vi "LJstreamUD read config.vi"(0 "Working Directory":path, 5 "filename":string="ljstreamud.cfg", 7 "ChP Default":string="0#!#1#!#2#!#3#!#4#!#5#!#6#!#7#!#8#!#9#!#10#!#11#!#12#!#13#!#14#!#15#!#") -> (1 "Data File Prefix":string="data", 2 "Scan Rate (Hz)":dbl=500.0 format="%.3f", 3 "Graph History":i32=1000 min=0, 4 "# Channels":i32=4, 6 "Disable Scaling":bool, 8 "Max File Size (Bytes)":i32=1048576, 9 "Write To File":bool, 10 "Channel Setup":T1={"+Ch"=["0", "1", "2", "3", "4", "5", "6", "7"], "-Ch"=["199", "199", "199", "199", "199", "199", "199", "199"], "Ranges"=[0, 0, 0, 0, 0, 0, 0, 0], "Scaling Equation"=["y=v0", "y=v1", "y=v2", "y=v3", "y=v4", "y=v5", "y=v6", "y=v7"], "Graph?"=[]} {"Ranges" items=["LJ_rgBIP10V", "LJ_rgBIP5V", "LJ_rgUNI5V", "LJ_rgUNI2P5V", "LJ_rgUNI1P25V", "LJ_rgBIP1V", "LJ_rgUNIP625V", "LJ_rgBIPP1V", "LJ_rgBIPP01V"]}, 12 "Interval (ms)":u32=500, 13 "Resolution":u8, 14 "SettlingFactor":u8, 15 "error out":errorcluster)   [LabVIEW 2021]
uses:
  <vilib>/Utility/config.llb/Read Key (String).vi
  <vilib>/Utility/config.llb/Read Key (U32).vi
  <vilib>/Utility/config.llb/Read Key (Double).vi
  <vilib>/Utility/config.llb/Read Key (I32).vi
  <vilib>/Utility/config.llb/Read Key (Boolean).vi
  <vilib>/Utility/config.llb/NI_LVConfig.lvlib
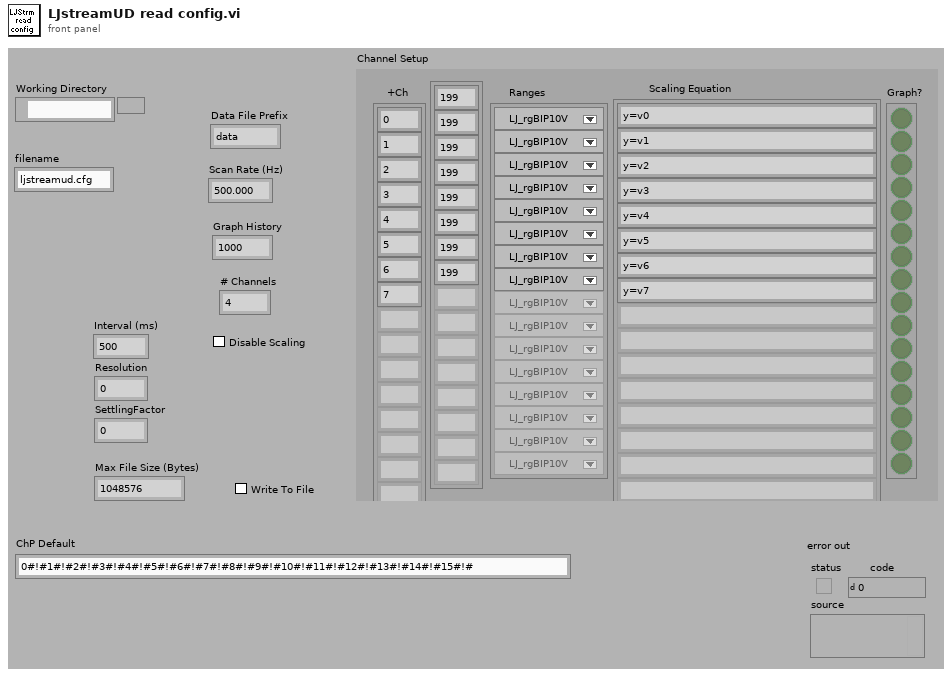
[diagram p1: front panel]
types:
  T1 = cluster{"+Ch":string[], "-Ch":string[], "Ranges":u16[], "Scaling Equation":string[], "Graph?":bool[]}
  T2 = typedef "NI_LVConfig.lvlib/Config Data RefNum.ctl" = refnum<k1>
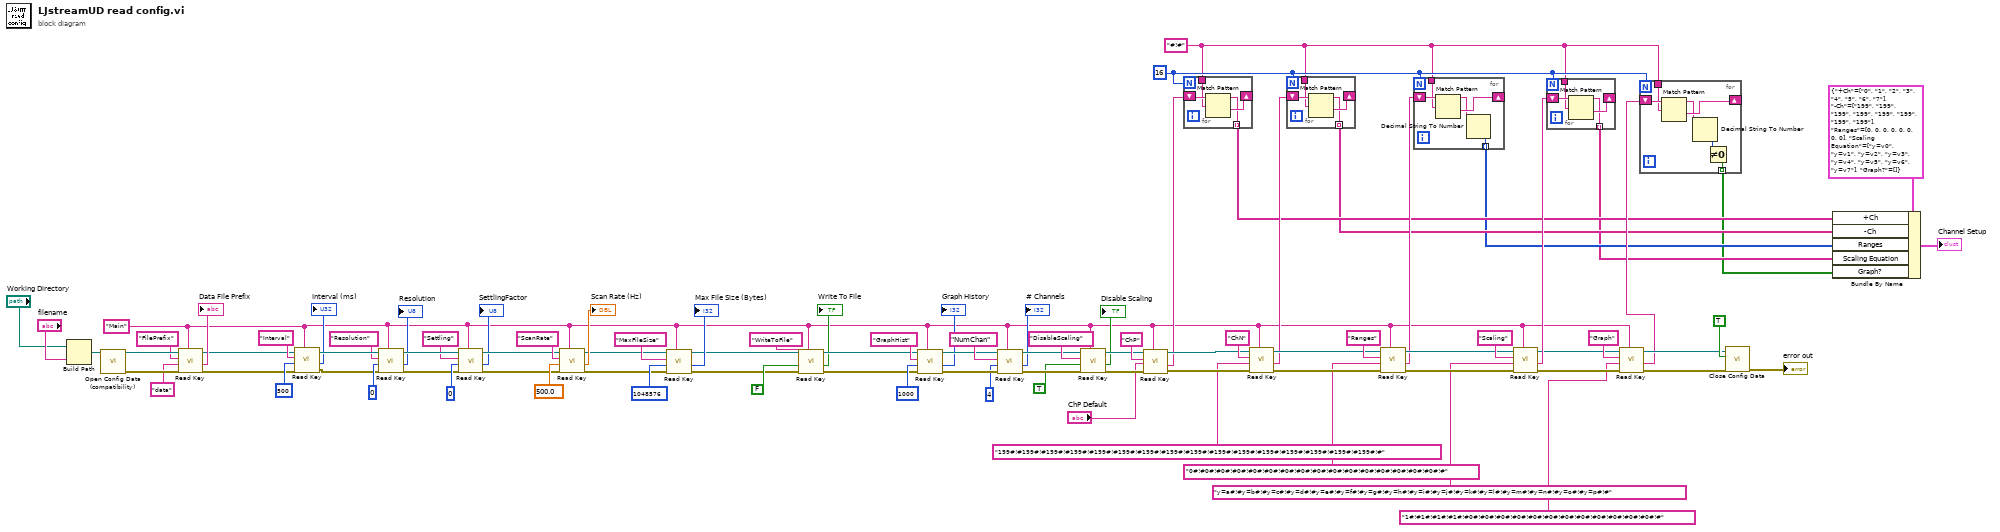
[diagram p0: block diagram]
diagram:
  w50 = 16
  w48 = "#!#" ("delimiter (Tab)")
  w1 = "Main" ("section")
  n1 = Build Path(base path="Working Directory", name or relative path="filename") -> (appended path=w91:path)
  n2 = call <vilib>:"Open Config Data (compatibility).vi"("configuration file path"=w91) -> ("error out"=w88:errorcluster, "refnum"=w89:T2)  [unwired: 8 in, 1 out]
  n3 = call-poly <vilib>:"Read Key.vi"("section"=w1, "error in (no error)"=w88, "default value"="data" ("Data File Prefix"), "key"="FilePrefix", "refnum"=w89) -> ("error out"=w22:errorcluster, "value"=→"Data File Prefix":string, "refnum out"=w20:T2)  [unwired: 3 in, 1 out]
  n4 = call-poly <vilib>:"Read Key.vi"("section"=w1, "error in (no error)"=w22, "default value"=u32 500 ("Scan Rate (Hz)"), "key"="Interval", "refnum"=w20) -> ("error out"=w27:errorcluster, "value"=→"Interval (ms)":u32, "refnum out"=w26:T2)  [unwired: 3 in, 1 out]
  n5 = call-poly <vilib>:"Read Key.vi"("section"=w1, "error in (no error)"=w27, "default value"=u8 0 ("Graph History"), "key"="Resolution", "refnum"=w26) -> ("error out"=w29:errorcluster, "value"=→"Resolution":u32, "refnum out"=w28:T2)  [unwired: 3 in, 1 out]
  n6 = call-poly <vilib>:"Read Key.vi"("section"=w1, "error in (no error)"=w29, "default value"=u8 0 ("# Channels"), "key"="Settling", "refnum"=w28) -> ("error out"=w21:errorcluster, "value"=→"SettlingFactor":u32, "refnum out"=w19:T2)  [unwired: 3 in, 1 out]
  n7 = call-poly <vilib>:"Read Key.vi"("section"=w1, "error in (no error)"=w21, "default value"=500.0 ("Scan Rate (Hz)"), "key"="ScanRate", "refnum"=w19) -> ("error out"=w12:errorcluster, "value"=→"Scan Rate (Hz)":dbl, "refnum out"=w11:T2)  [unwired: 3 in, 1 out]
  n8 = call-poly <vilib>:"Read Key.vi"("section"=w1, "error in (no error)"=w12, "default value"=1048576 ("Graph History"), "key"="MaxFileSize", "refnum"=w11) -> ("error out"=w5:errorcluster, "value"=→"Max File Size (Bytes)":i32, "refnum out"=w6:T2)  [unwired: 3 in, 1 out]
  n9 = call-poly <vilib>:"Read Key.vi"("section"=w1, "error in (no error)"=w5, "default value"=FALSE, "key"="WriteToFile", "refnum"=w6) -> ("error out"=w3:errorcluster, "value"=→"Write To File":bool, "refnum out"=w4:T2)  [unwired: 3 in, 1 out]
  n10 = call-poly <vilib>:"Read Key.vi"("section"=w1, "error in (no error)"=w3, "default value"=1000 ("Graph History"), "key"="GraphHist", "refnum"=w4) -> ("error out"=w83:errorcluster, "value"=→"Graph History":i32, "refnum out"=w84:T2)  [unwired: 3 in, 1 out]
  n11 = call-poly <vilib>:"Read Key.vi"("section"=w1, "error in (no error)"=w83, "default value"=4 ("# Channels"), "key"="NumChan", "refnum"=w84) -> ("error out"=w58:errorcluster, "value"=→"# Channels":i32, "refnum out"=w59:T2)  [unwired: 3 in, 1 out]
  n12 = call-poly <vilib>:"Read Key.vi"("section"=w1, "error in (no error)"=w58, "default value"=TRUE, "key"="DisableScaling", "refnum"=w59) -> ("error out"=w56:errorcluster, "value"=→"Disable Scaling":bool, "refnum out"=w55:T2)  [unwired: 3 in, 1 out]
  n13 = call-poly <vilib>:"Read Key.vi"("section"=w1, "error in (no error)"=w56, "default value"="ChP Default", "key"="ChP", "refnum"=w55) -> ("error out"=w78:errorcluster, "value"=w64:string, "refnum out"=w79:T2)  [unwired: 3 in, 1 out]
  n14 = for {
    N: w50 -> [_]
    shift-right: [w94] -> _
    shift-left: w64 -> [w96]
    tunnel: w48 -> [w95]
    tunnel: [w93] -> w38 mode=indexing
    n15 = Match Pattern(string=w96, regular expression=w95) -> (before substring=w93:string, after substring=w94:string)  [unwired: 1 in, 2 out]
  }
  n16 = call-poly <vilib>:"Read Key.vi"("section"=w1, "error in (no error)"=w78, "default value"="199#!#199#!#199#!#199#!#199#!#199#!#199#!#199#!#199#!#199#!#199#!#199#!#199#!#199#!#199#!#199#!#" ("Data File Prefix"), "key"="ChN", "refnum"=w79) -> ("error out"=w77:errorcluster, "value"=w63:string, "refnum out"=w76:T2)  [unwired: 3 in, 1 out]
  n17 = for {
    N: w50 -> [_]
    shift-right: [w98] -> _
    shift-left: w63 -> [w100]
    tunnel: w48 -> [w99]
    tunnel: [w97] -> w37 mode=indexing
    n18 = Match Pattern(string=w100, regular expression=w99) -> (before substring=w97:string, after substring=w98:string)  [unwired: 1 in, 2 out]
  }
  n19 = call-poly <vilib>:"Read Key.vi"("section"=w1, "error in (no error)"=w77, "default value"="0#!#0#!#0#!#0#!#0#!#0#!#0#!#0#!#0#!#0#!#0#!#0#!#0#!#0#!#0#!#0#!#" ("Data File Prefix"), "key"="Ranges", "refnum"=w76) -> ("error out"=w74:errorcluster, "value"=w62:string, "refnum out"=w73:T2)  [unwired: 3 in, 1 out]
  n20 = for {
    N: w50 -> [_]
    shift-right: [w103] -> _
    shift-left: w62 -> [w105]
    tunnel: w48 -> [w104]
    tunnel: [w101] -> w36 mode=indexing
    n21 = Match Pattern(string=w105, regular expression=w104) -> (before substring=w102:string, after substring=w103:string)  [unwired: 1 in, 2 out]
    n22 = Decimal String To Number(string=w102) -> (number=w101:i32)  [unwired: 2 in, 1 out]
  }
  n23 = call-poly <vilib>:"Read Key.vi"("section"=w1, "error in (no error)"=w74, "default value"="y=a#!#y=b#!#y=c#!#y=d#!#y=e#!#y=f#!#y=g#!#y=h#!#y=i#!#y=j#!#y=k#!#y=l#!#y=m#!#y=n#!#y=o#!#y=p#!#" ("Data File Prefix"), "key"="Scaling", "refnum"=w73) -> ("error out"=w53:errorcluster, "value"=w61:string, "refnum out"=w46:T2)  [unwired: 3 in, 1 out]
  n24 = for {
    N: w50 -> [_]
    shift-right: [w107] -> _
    shift-left: w61 -> [w109]
    tunnel: w48 -> [w108]
    tunnel: [w106] -> w35 mode=indexing
    n25 = Match Pattern(string=w109, regular expression=w108) -> (before substring=w106:string, after substring=w107:string)  [unwired: 1 in, 2 out]
  }
  n26 = call-poly <vilib>:"Read Key.vi"("section"=w1, "error in (no error)"=w53, "default value"="1#!#1#!#1#!#1#!#0#!#0#!#0#!#0#!#0#!#0#!#0#!#0#!#0#!#0#!#0#!#0#!#" ("Data File Prefix"), "key"="Graph", "refnum"=w46) -> ("error out"=w52:errorcluster, "value"=w49:string, "refnum out"=w51:T2)  [unwired: 3 in, 1 out]
  n27 = for {
    N: w50 -> [_]
    shift-right: [w113] -> _
    shift-left: w49 -> [w115]
    tunnel: w48 -> [w114]
    tunnel: [w110] -> w34 mode=indexing
    n28 = Match Pattern(string=w115, regular expression=w114) -> (before substring=w112:string, after substring=w113:string)  [unwired: 1 in, 2 out]
    n29 = Decimal String To Number(string=w112) -> (number=w111:i32)  [unwired: 2 in, 1 out]
    n30 = Not Equal To 0?(x=w111) -> (x != 0?=w110:bool)
  }
  n31 = call <vilib>:"Close Config Data.vi"("error in (no error)"=w52, "write file if changed (T)"=TRUE ("write configuration file? (F)"), "refnum"=w51) -> ("error out"=→"error out":errorcluster)  [unwired: 7 in, 1 out]
  n32 = Bundle By Name(cluster=T1 {"+Ch"=["0", "1", "2", "3", "4", "5", "6", "7"], "-Ch"=["199", "199", "199", "199", "199", "199", "199", "199"], "Ranges"=[0, 0, 0, 0, 0, 0, 0, 0], "Scaling Equation"=["y=v0", "y=v1", "y=v2", "y=v3", "y=v4", "y=v5", "y=v6", "y=v7"], "Graph?"=[]} ("Channel Setup"), "+Ch"=w38, "-Ch"=w37, "Ranges"=w36, "Scaling Equation"=w35, "Graph?"=w34) -> (→"Channel Setup":T1)
